vi "Hokuyo Two.vi"() -> ()   [LabVIEW 2014]
uses:
  <instrlib>/Hokuyo URG Series/Public/Initialize-Standard.vi
  <instrlib>/Hokuyo URG Series/Hokuyo URG Series.lvlib
panel:
  out "Blinky LIDAR  Running":bool
  in  "polar attributes (hidden)":T1={"maximum"=30000.0, "minimum"=0.0, "clip to min"=FALSE, "log?(F)"=TRUE, "grid color"=6710886, "plot color"=65280, "fmt and prec"={"format"=enum."Decimal", "precision"=0}, "visible section"=8} {"minimum" format="%0.2f"; "maximum" format="%0.2f"}
  in  "VISA resource name":refnum<visa-resource-name>="COM3"
  in  "Stop":bool
  out "Data Aquired":picture
  in  "Grid Color":u32(colorbox)=11776947
  in  "Plot Color":u32(colorbox)=14422272
  in  "Max (m)":dbl=1.0
  in  "End Point":dbl=33.0
  in  "Start Point":dbl=-50.0
  in  "Cluster Count":dbl=1.0
  in  "Encoding Width":u16(ring)=3 items=["2 Byte"=2, "3 Byte"=3]
  # "click here to run"
  # "Hokuyo LIDAR Example"
  # "Plot in mm"
  # "start at-50"
  # "start at 33"
  # "Start with 1.0 m"
  # "Hokuyo plugged in?"
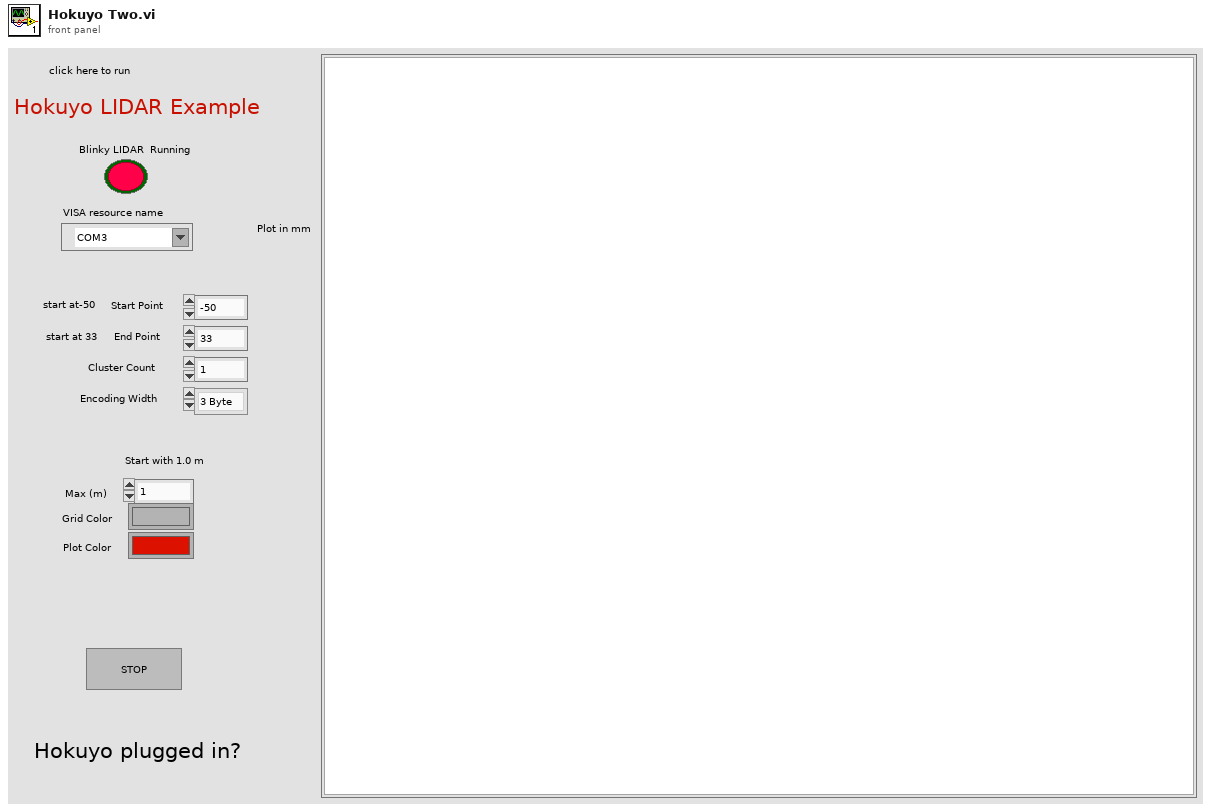
[diagram p1: front panel]
types:
  T1 = cluster{"maximum":dbl, "minimum":dbl, "clip to min":bool, "log?(F)":bool, "grid color":u32, "plot color":u32, "fmt and prec":cluster{"format":enum8{"Decimal", "Scientific", "Engineering", "Binary", "Octal", "Hex"}, "precision":u8}, "visible section":u16}
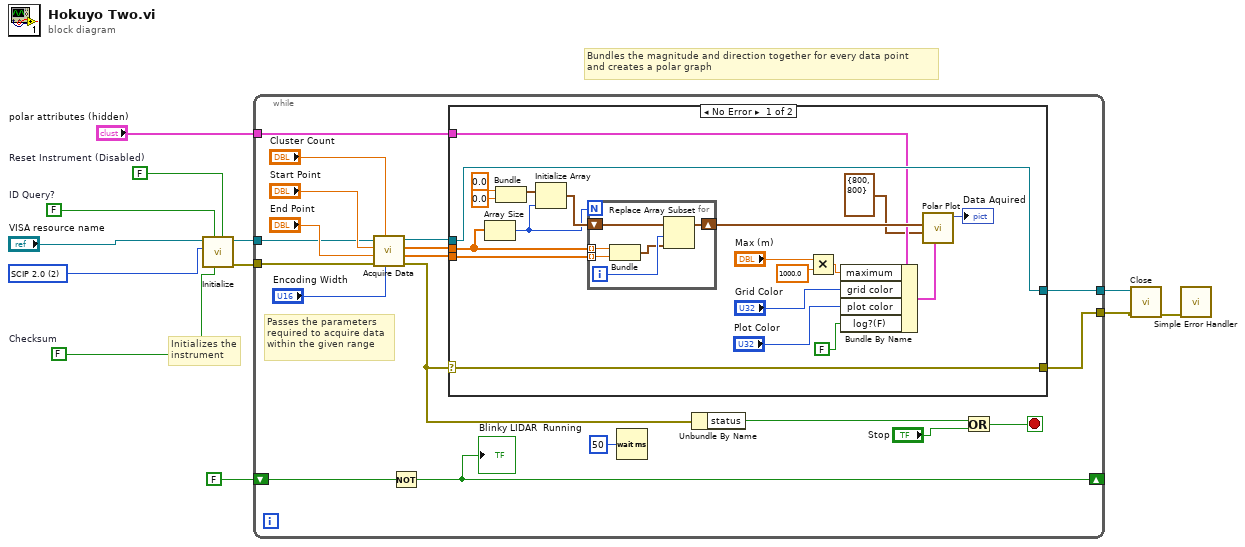
[diagram p0: block diagram]
diagram:
  w10 = FALSE  # Checksum
  w8 = FALSE  # ID Query?
  w6 = u32 2 items=["Convert to Latest", "SCIP 1.1", "SCIP 2.0"] ("Protocol")
  w7 = FALSE  # Reset Instrument (Disabled)
  # "Bundles the magnitude and direction together for every data point\nand creates a polar graph"
  # "Initializes the instrument"
  n1 = call-poly <instrlib>:"Initialize.vi"("Reset? (F: No)"=w7, "Checksum (Disabled)"=w10, "ID Query? (Enabled)"=w8, "Protocol (2: SCIP 2.0)"=w6, "VISA resource name"="VISA resource name") -> ("error out"=w3:errorcluster, "VISA resource name out"=w4:refnum<visa-resource-name>)  [unwired: 5 in]
  n2 = while {
    tunnel: w4 -> [w19]
    tunnel: [w31] -> w12
    tunnel: [w30] -> w5
    tunnel: w3 -> [w18]
    tunnel: "polar attributes (hidden)" -> [w17]
    shift-right: [w13] -> _
    shift-left: FALSE -> [w14]
    stop <- w27 stop-if-true
    # "Passes the parameters\nrequired to acquire data\nwithin the given range"
    n3 = call <instrlib>:"Acquire Data.vi"("Data Encoding Width (3 Byte)"="Encoding Width", "Cluster Count (1)"="Cluster Count", "error in (no error)"=w18, "End Point (120°)"="End Point", "Start Point (-120°)"="Start Point", "VISA resource name"=w19) -> ("error out"=w23:errorcluster, "Direction"=w24:dbl[], "Magnitude"=w25:dbl[], "VISA resource name out"=w26:refnum<visa-resource-name>)  [unwired: 2 in]
    n4 = Not(x=w14) -> (.not. x?=w13:bool)
    "Blinky LIDAR  Running" <- w13
    n5 = case shown="No Error" w23 {
      selector: w23 -> [w49 w59]
      tunnel: [w49 w59] -> w31
      tunnel: w26 -> [w50 w58]
      tunnel: [w50 w58] -> w30
      tunnel: w25 -> [w44 _]
      tunnel: w24 -> [w43 _]
      tunnel: w17 -> [w39 _]
      frame No Error {
        n6 = Array Size(array=w44) -> (size(s)=w42:i32)
        n7 = Bundle(0.0, 0.0) -> (w46:cluster{dbl, dbl})  [unwired: 1 in]
        n8 = Initialize Array(w46, w42) -> (w45:cluster{dbl, dbl}[])
        n9 = for {
          N: w42 -> [_]
          shift-right: [w53] -> w41
          shift-left: w45 -> [w54]
          tunnel: w44 -> [w57] mode=indexing
          tunnel: w43 -> [w56] mode=indexing
          i -> [w55]
          n10 = Bundle(w57, w56) -> (w52:cluster{dbl, dbl})  [unwired: 1 in]
          n11 = Replace Array Subset(array=w54, new element=w52, index=w55) -> (w53:cluster{dbl, dbl}[])
        }
        n12 = Multiply(x="Max (m)", y=1000.0) -> (x*y=w35:dbl)
        n13 = Bundle By Name(cluster=w39, "maximum"=w35, "grid color"="Grid Color", "plot color"="Plot Color", "log?(F)"=FALSE) -> (w40:T1)
        n14 = call <vilib>:"Polar Plot.vi"("polar attributes"=w40, "dimensions (w,h)"=cluster{"width":i16, "height":i16} {"width"=800, "height"=800}, "data array [mag, phase (deg)]"=w41) -> ("new picture"=→"Data Aquired":picture)  [unwired: 8 in]
      }
      frame Error {
      }
    }
    n15 = Wait (ms)(milliseconds to wait=u32 50) -> ()  [unwired: 1 out]
    n16 = Unbundle By Name(w23) -> ("status"=w29:bool)
    n17 = Or(x=w29, y="Stop") -> (x .or. y?=w27:bool)
  }
  n18 = call <instrlib>:"Close.vi"("error in (no error)"=w12, "VISA resource name"=w5) -> ("error out"=w9:errorcluster)  [unwired: 9 in]
  n19 = call <vilib>:"Simple Error Handler.vi"("error in (no error)"=w9) -> ()  [unwired: 4 in, 5 out]
